vi "Grap.vi"(8 "error in (no error)":errorcluster, 11 "CCD monitor in":refnum<class "CCD monitor.lvclass">) -> (0 "error out":errorcluster, 3 "CCD monitor out":refnum<class "CCD monitor.lvclass">)   [LabVIEW 2016, in "CCD monitor.lvlib" / "CCD monitor.lvclass"]
uses:
  <userlib>/Common Components/Hardware/Abstract System/Monitor/CCD monitor.lvclass
  <userlib>/Common Components/Hardware/Abstract System/Monitor/CCD monitor.lvclass/CCD monitor.ctl
  <userlib>/Common Components/Hardware/CCD/CCD/CCD.lvclass/CCD.ctl
  <userlib>/Common Components/Hardware/CCD/CCD/Read New Image.vi
  <userlib>/Common Components/Hardware/CCD/CCD/Write New Image.vi
  <userlib>/Common Components/Hardware/CCD/CCD/CCD.lvclass
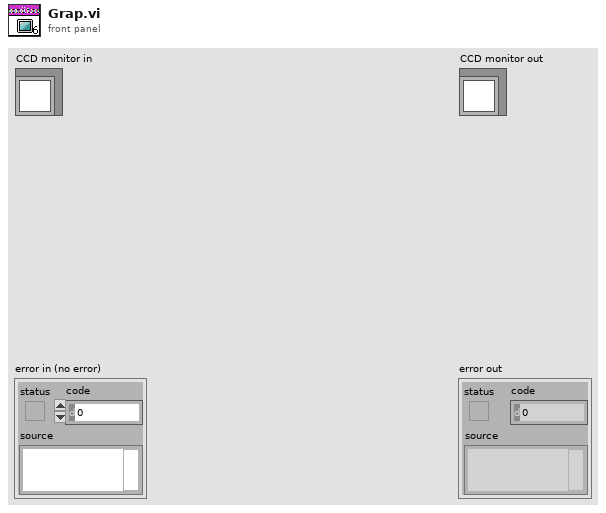
[diagram p1: front panel]
types:
  T1 = typedef "IMAQ Image.ctl" = refnum<image>
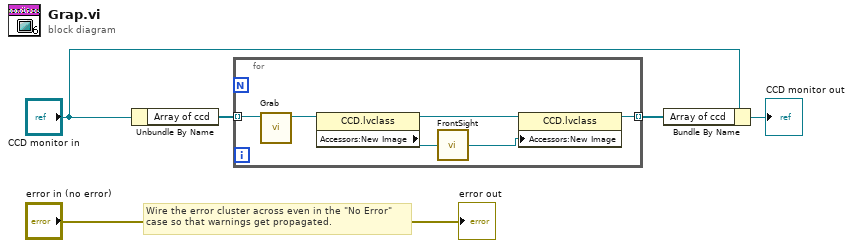
[diagram p0: block diagram]
diagram:
  # "Wire the error cluster across even in the \"No Error\"\ncase so that warnings get propagated."
  n1 = Unbundle By Name("CCD monitor in") -> ("Array of ccd"=w4:refnum<class "CCD.lvclass">[])
  n2 = for {
    tunnel: w4 -> [w11] mode=indexing
    tunnel: [w7] -> w2 mode=indexing
    n3 = call-dynamic "Grab.vi"("CCD in"=w11) -> ("CCD out"=w8:refnum<class "CCD.lvclass">)  [unwired: 9 in, 1 out]
    n4 = property class="CCD.lvclass"(reference=w8) -> (reference out=w6:refnum<class "CCD.lvclass">, "Accessors:New Image"=w10:T1)  [unwired: 1 in, 1 out]
    n5 = call <userlib>:"FrontSight.vi"("IMAQImage"=w10) -> ("Image Out"=w9:T1)
    n6 = property class="CCD.lvclass"(reference=w6, "Accessors:New Image"=w9) -> (reference out=w7:refnum<class "CCD.lvclass">)  [unwired: 1 in, 1 out]
  }
  n7 = Bundle By Name(cluster="CCD monitor in", "Array of ccd"=w2) -> (→"CCD monitor out":refnum<class "CCD monitor.lvclass">)
  "error out" <- "error in (no error)"
